vi "test Get Attribute as String.vi"(11 "Test Case In":refnum<class "Test Config From Excel Table.lvclass">) -> (0 "error out":errorcluster, 3 "Test Case Out":refnum<class "Test Config From Excel Table.lvclass">)   [LabVIEW 2020, in "Test Config From Excel Table.lvclass"]
uses:
  Test Config From Excel Table.lvclass
  C:/Program Files/National Instruments/LabVIEW 2025/vi.lib/Astemes/LUnit/Test Case.lvclass
  Source/Config from Excel Table/Config from Excel Table.lvclass
  <vilib>/Astemes/LUnit/Test Case.lvclass/Test Case.ctl
  Test Config From Excel Table.lvclass/Test Config From Excel Table.ctl
  <vilib>/Astemes/LUnit/Test Case.lvclass
  <vilib>/Peter/Open Xml/Source/Open Xml.lvlib
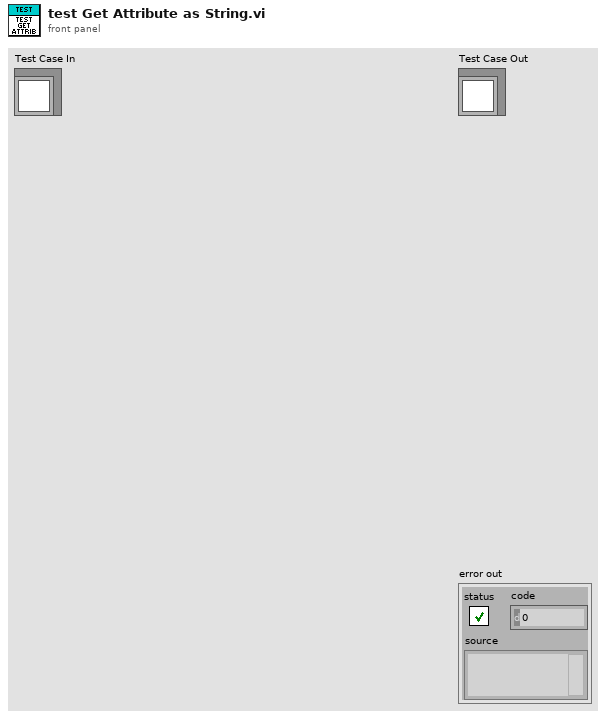
[diagram p1: front panel]
types:
  T1 = cluster{"Sheet Name":string, "Name":string, "Display Name":string, "Range or Cell Address":string}
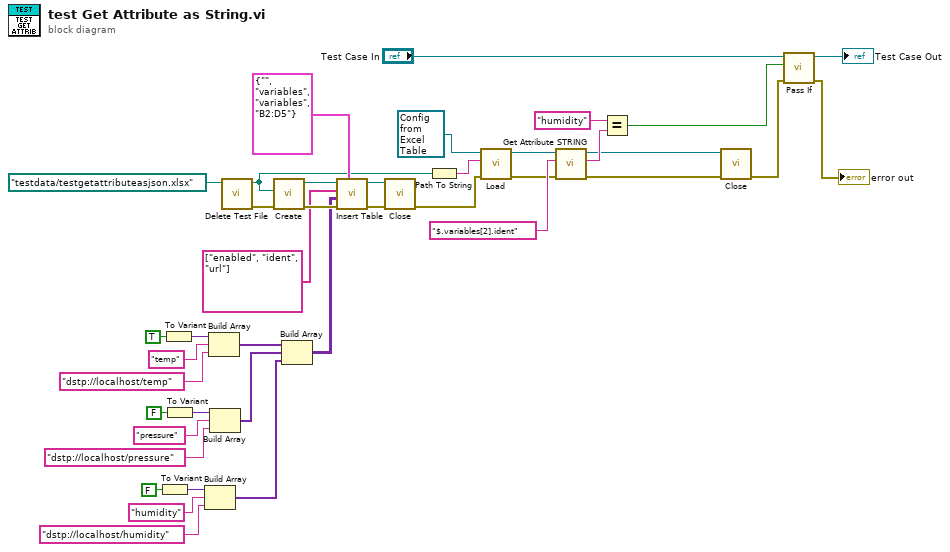
[diagram p0: block diagram]
diagram:
  n1 = To Variant(anything=FALSE) -> (Variant=w12:variant)
  n2 = To Variant(anything=TRUE) -> (Variant=w21:variant)
  n3 = To Variant(anything=FALSE) -> (Variant=w15:variant)
  n4 = Build Array(w12, "humidity", "dstp://localhost/humidity") -> (w8:variant[])
  n5 = Build Array(w21, "temp", "dstp://localhost/temp") -> (w18:variant[])
  n6 = Build Array(w15, "pressure", "dstp://localhost/pressure") -> (w9:variant[])
  n7 = call "Delete Test File.vi"("name or relative path"=path "testdata/testgetattributeasjson.xlsx") -> ("error out"=w26:errorcluster, "deleted path"=w2:path)  [unwired: 9 in]
  n8 = call <vilib>:"Create.vi"("error in"=w26, "Path"=w2) -> ("error out"=w25:errorcluster, "SpreadsheetDoc"=w6:refnum<k24>)  [unwired: 8 in]
  n9 = Build Array(w18, w9, w8) -> (w7:variant[][])
  n10 = call <vilib>:"Insert Table.vi"("Location"=T1 {"Sheet Name"="", "Name"="variables", "Display Name"="variables", "Range or Cell Address"="B2:D5"}, "error in"=w25, "Cell Values"=w7, "Header Names"=string[] ["enabled", "ident", "url"], "SpreadsheetDoc in"=w6) -> ("error out"=w5:errorcluster, "SpreadsheetDoc out"=w4:refnum<k24>)  [unwired: 5 in]
  n11 = call <vilib>:"Close.vi"("error in"=w5, "SpreadsheetDoc"=w4) -> ("error out"=w1:errorcluster)  [unwired: 9 in]
  n12 = Path To String(path=w2) -> (string=w36:string)
  n13 = call-dynamic "Load.vi"("error in"=w1, "Source"=w36, "Config from Excel Table in"=refnum<class "Config from Excel Table.lvclass"> refnum ("Config from EXCEL Table.lvclass")) -> ("error out"=w27:errorcluster, "Config from Excel Table out"=w28:refnum<class "Config from Excel Table.lvclass">)  [unwired: 7 in]
  n14 = call-dynamic "Get Attribute STRING.vi"("error in"=w27, "Attribute"="$.variables[2].ident", "Config from Excel Table in"=w28) -> ("error out"=w30:errorcluster, "Value"=w33:string, "Config from Excel Table out"=w31:refnum<class "Config from Excel Table.lvclass">)  [unwired: 6 in]
  n15 = Equal?(x="humidity" ("Value"), y=w33) -> (x = y?=w32:bool)
  n16 = call-dynamic <vilib>:"Close.vi"("error in"=w30, "Config from Excel Table in"=w31) -> ("error out"=w29:errorcluster)  [unwired: 8 in, 1 out]
  n17 = call <vilib>:"Pass If.vi"("error in (no error)"=w29, "Pass?"=w32, "LUnit Test Case In"="Test Case In") -> ("error out"=→"error out":errorcluster, "LUnit Test Case Out"=→"Test Case Out":refnum<class "Test Config From Excel Table.lvclass">)  [unwired: 7 in]
